vi "Add Module via VI Reference.vi"(8 "error in (no error)":errorcluster, 9 "Module Name":string, 10 "VI Ref":refnum<vi>, 11 "SLL Subpanel Manager in":refnum<class "SLL Subpanel Manager.lvclass">) -> (0 "error out":errorcluster, 3 "SLL Subpanel Manager out":refnum<class "SLL Subpanel Manager.lvclass">)   [LabVIEW 2016, in "SLL Subpanel Manager.lvclass"]
uses:
  SLL Subpanel Manager.lvclass
  SLL Subpanel Manager.lvclass/SLL Subpanel Manager.ctl
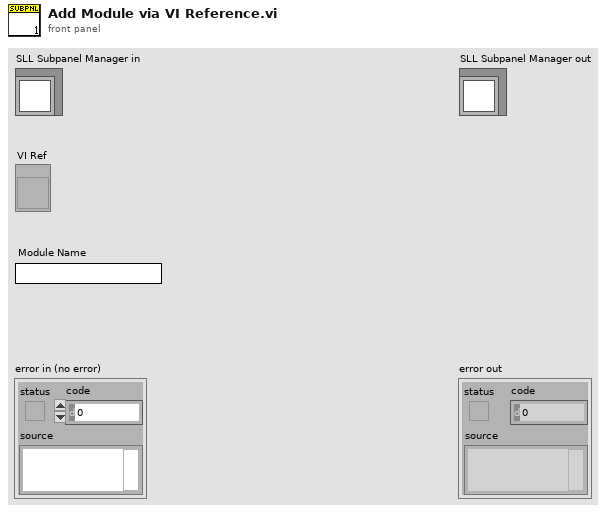
[diagram p1: front panel]
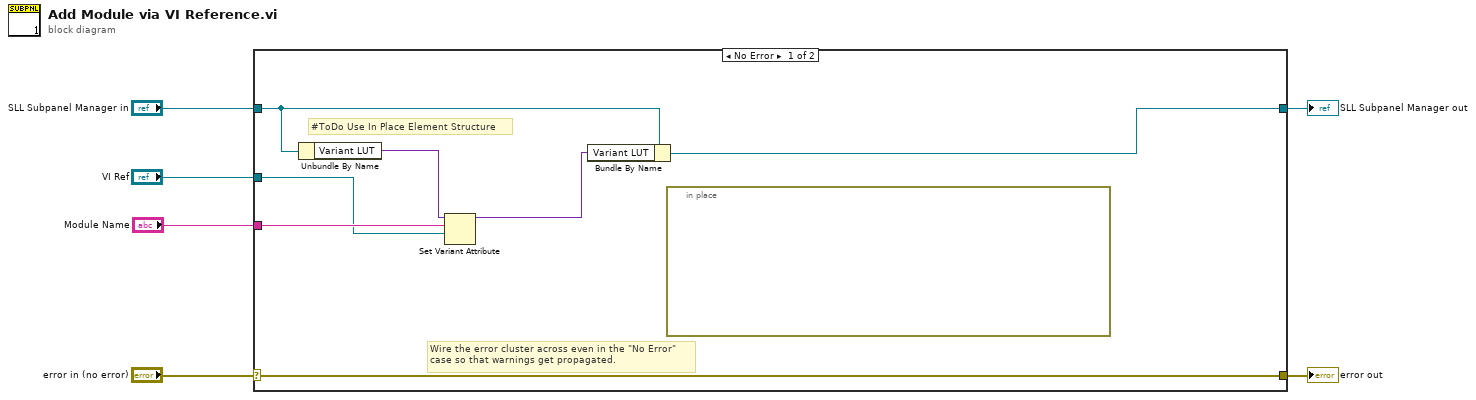
[diagram p0: block diagram]
diagram:
  n1 = case shown="No Error" "error in (no error)" {
    selector: "error in (no error)" -> [w13 w15]
    tunnel: [w13 w15] -> w5
    tunnel: [w8 w14] -> w3
    tunnel: "SLL Subpanel Manager in" -> [w9 w14]
    tunnel: "Module Name" -> [w11 _]
    tunnel: "VI Ref" -> [w10 _]
    frame No Error {
      # "#ToDo Use In Place Element Structure"
      # "Wire the error cluster across even in the \"No Error\"\ncase so that warnings get propagated."
      n2 = Unbundle By Name(w9) -> ("Variant LUT"=w12:variant)
      n3 = Set Variant Attribute(Variant=w12, name=w11, value=w10) -> (Variant out=w7:variant)  [unwired: 1 in, 2 out]
      n4 = Bundle By Name(cluster=w9, "Variant LUT"=w7) -> (w8:refnum<class "SLL Subpanel Manager.lvclass">)
      n5 = in-place {
      }
    }
    frame Error {
    }
  }
  "error out" <- w5
  "SLL Subpanel Manager out" <- w3
